vi "ReportEnd.vi"(6 "文件重命名":bool, 7 "产品型号":string, 8 "error in (no error)":errorcluster caption="错误输入（无错误）", 10 "文件名称":string, 11 "report in":refnum<class "NI_report.lvclass"> caption="报表输入") -> (0 "error out":errorcluster caption="错误输出")   [LabVIEW 2020]
uses:
  <vilib>/Utility/NIReport.llb/NI_report.lvclass
panel:
  out "添加的路径":path
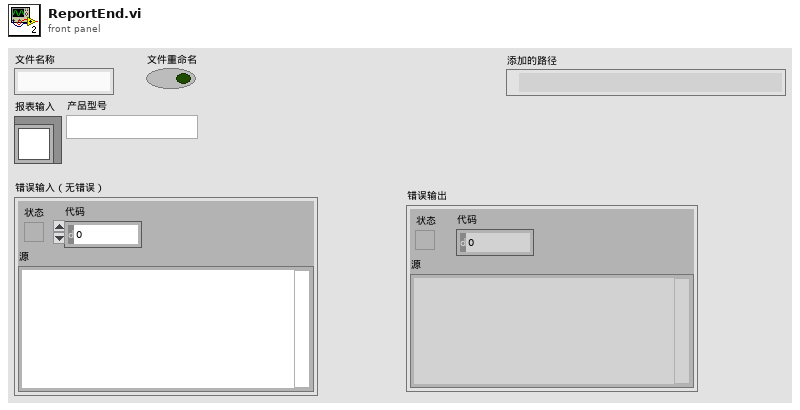
[diagram p1: front panel]
types:
  T1 = cluster{"Italic":enum16{"Italic Unchanged", "Italic On", "Italic Off"}, "Strike Through":enum16{"Strike Through Unchanged", "Strike Through On", "Strike Through Off"}, "Underline":enum16{"Underline Unchanged", "Underline On", "Underline Off"}, "Bold":enum16{"Bold Unchanged", "Bold On", "Bold Off"}}
  T2 = cluster{"Charset (-1)":i16, "Weight (-1)":i16, "Name":string, "Size":string}
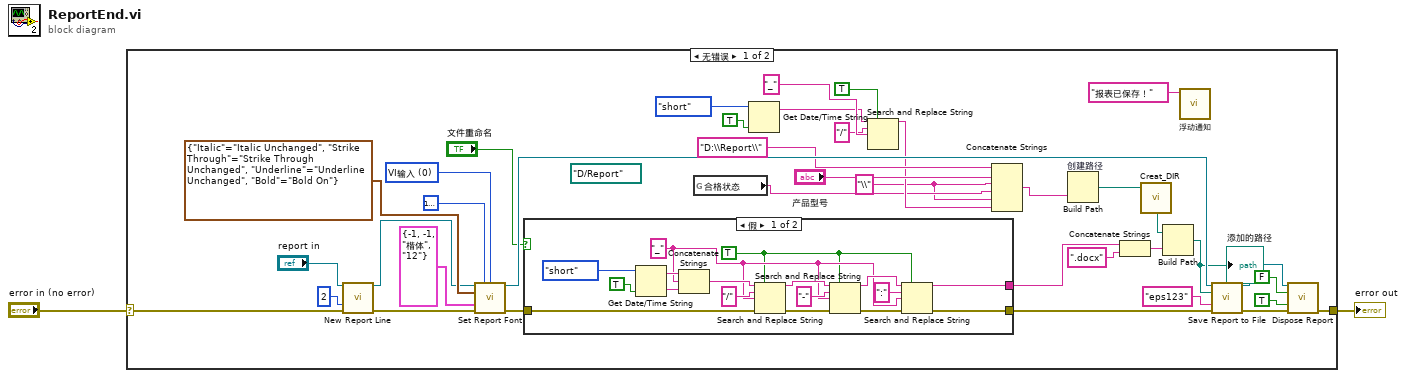
[diagram p0: block diagram]
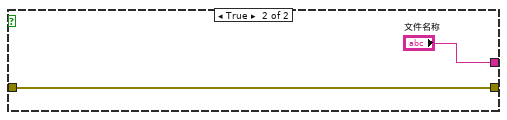
[diagram p2: hidden frame]
diagram:
  n1 = case shown="无错误" "error in (no error)" {
    selector: "error in (no error)" -> [w25 w60]
    tunnel: [w24 w60] -> w1
    frame No Error {
      w3 = "\\" ("搜索字符串")
      w35 = u16 0 items=["VI输入", "字体对话框"] ("font settings source")
      (unwired) path "D:/Report" ("report file path")
      n2 = call-dynamic "New Report Line.vi"("report in"="report in", "number of lines (1)"=2, "error in (no error)"=w25) -> ("report out"=w32:refnum<class "NI_report.lvclass">, "error out"=w31:errorcluster)  [unwired: 11 in]
      n3 = call-dynamic "Set Report Font.vi"("report in"=w32, "text color (unchanged)"=u32 16777224, "font settings source (VI Inputs)"=w35, "text options"=T1 {"Italic"=enum."Italic Unchanged", "Strike Through"=enum."Strike Through Unchanged", "Underline"=enum."Underline Unchanged", "Bold"=enum."Bold On"}, "font settings"=T2 {"Charset (-1)"=-1, "Weight (-1)"=-1, "Name"="楷体", "Size"="12"}, "error in (no error)"=w31) -> ("report out"=w28:refnum<class "NI_report.lvclass">, "error out"=w27:errorcluster)  [unwired: 7 in, 1 out]
      n4 = case shown="假" "文件重命名" {
        tunnel: [w52 "文件名称"] -> w22
        tunnel: w27 -> [w44 w59]
        tunnel: [w41 w59] -> w26
        frame False {
          w46 = TRUE ("替换全部？(F)")
          w47 = "_" ("替换字符串(\"\")")
          n5 = Get Date/Time String(date format (0)=enum16{"short", "long", "abbreviated"}."short" ("日期格式(0)"), want seconds? (F)=TRUE ("需要秒？(F)")) -> (date string=w57:string, time string=w53:string)  [unwired: 1 in]
          n6 = Concatenate Strings(w57, w47, w53) -> (w50:string)
          n7 = Search and Replace String(replace all?=w46, input string=w50, search string="/" ("搜索字符串"), replace string=w47, error in=w44) -> (result string=w49:string, error out=w43:errorcluster)  [unwired: 3 in, 2 out]
          n8 = Search and Replace String(replace all?=w46, input string=w49, search string="-" ("搜索字符串"), replace string=w47, error in=w43) -> (result string=w55:string, error out=w42:errorcluster)  [unwired: 3 in, 2 out]
          n9 = Search and Replace String(replace all?=w46, input string=w55, search string=":" ("搜索字符串"), replace string=w47, error in=w42) -> (result string=w52:string, error out=w41:errorcluster)  [unwired: 3 in, 2 out]
        }
        frame True {
        }
      }
      n10 = global read "检测结果.vi" "合格状态"() -> (w4:string)
      n11 = Get Date/Time String(date format (0)=enum16{"short", "long", "abbreviated"}."short" ("日期格式(0)"), want seconds? (F)=TRUE ("需要秒？(F)")) -> (date string=w10:string)  [unwired: 1 in, 1 out]
      n12 = Search and Replace String(replace all?=TRUE ("替换全部？(F)"), input string=w10, search string="/" ("搜索字符串"), replace string="_" ("替换字符串(\"\")")) -> (result string=w7:string)  [unwired: 4 in, 3 out]
      n13 = Concatenate Strings("D:\\Report\\" ("字符串"), "产品型号", w3, w4, w3, w7) -> (w6:string)
      n14 = Build Path "创建路径"(name or relative path=w6) -> (appended path=w5:path)  [unwired: 1 in]
      n15 = Concatenate Strings(w22, ".docx" ("字符串")) -> (w21:string)
      n16 = call "Creat_DIR.vi"("path"=w5) -> ("created path"=w17:path)  [unwired: 10 in]
      n17 = Build Path(base path=w17, name or relative path=w21) -> (appended path=w16:path)
      "添加的路径" <- w16
      n18 = call "浮动通知.vi"("通知内容"="报表已保存！" ("Status")) -> ()  [unwired: 11 in]
      n19 = call-dynamic "Save Report to File.vi"("report in"=w28, "report file path"=w16, "password (\"\")"="eps123" ("password (\"\")"), "error in (no error)"=w26) -> ("report out"=w40:refnum<class "NI_report.lvclass">, "error out"=w39:errorcluster)  [unwired: 10 in]
      n20 = call-dynamic "Dispose Report.vi"("report in"=w40, "wait until printing completed? (T)"=FALSE, "save changes? (F)"=TRUE, "error in (no error)"=w39) -> ("error out"=w24:errorcluster)  [unwired: 11 in]
    }
    frame Error {
    }
  }
  "error out" <- w1
